vi "main.vi"() -> ()   [LabVIEW 2015]
panel:
  out "After":dbl
  out "Before":dbl
  out "String":string
  in  "s":bool
  out "F":dbl
  in  "C":dbl
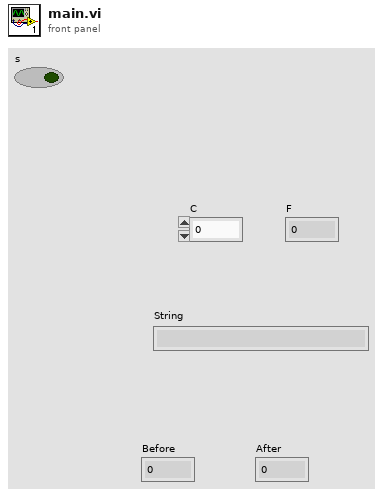
[diagram p1: front panel]
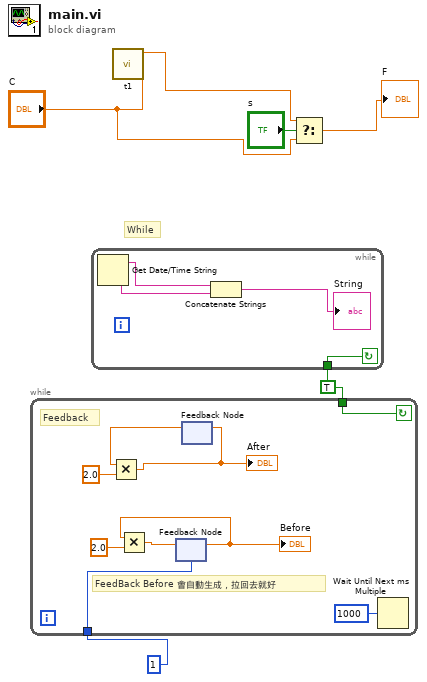
[diagram p0: block diagram]
diagram:
  w2 = TRUE
  # "While"
  n1 = while {
    tunnel: w2 -> [w15]
    tunnel: 1 -> [w7]
    stop <- w15 continue-if-true
    # "FeedBack Before 會自動生成，拉回去就好"
    # "Feedback"
    n2 = feedback #1(w7) -> (w8:dbl)
    "Before" <- w8
    n3 = Multiply(x=w8, y=2.0) -> (x*y=w9:dbl)
    n4 = feedback-in #1(w9) -> ()
    n5 = feedback #2() -> (w10:dbl)  [unwired: 1 in]
    n6 = Multiply(x=w10, y=2.0) -> (x*y=w11:dbl)
    "After" <- w11
    n7 = feedback-in #2(w11) -> ()
    n8 = Wait Until Next ms Multiple(millisecond multiple=u32 1000) -> ()  [unwired: 1 out]
  }
  n9 = while {
    tunnel: w2 -> [w19]
    stop <- w19 continue-if-true
    n10 = Get Date/Time String() -> (date string=w18:string, time string=w17:string)  [unwired: 3 in]
    n11 = Concatenate Strings(w18, w17) -> (→"String":string)
  }
  n12 = call "t1.vi"("C"="C") -> ("Numeric"=w6:dbl)  [unwired: 10 in]
  n13 = Select(t=w6, s="s", f="C") -> (s? t:f=→"F":dbl)
